vi "test Subset Pointer.vi"(8 "error in (no error)":errorcluster, 11 "TestCase in":refnum<class "Lifecycle Tests.lvclass">) -> (0 "error out":errorcluster, 3 "TestCase out":refnum<class "Lifecycle Tests.lvclass">)   [LabVIEW 2017, in "Pointer Tests.lvlib" / "Lifecycle Tests.lvclass"]
uses:
  Lifecycle Tests.lvclass
  Source/Classes/Pointer/Public/New/New (4B).vi
  Source/Classes/Pointer/Public/Write/Write (1D I32).vi
  Source/Classes/Pointer/Public/Read/Read (0D I32).vi
  Source/Classes/Pointer/Public/Write/Write (0D I32).vi
  <vilib>/addons/_JKI Toolkits/VI Tester/TestCase.llb/TestCase.lvclass
  Source/Classes/Pointer/Pointer.lvclass
  C:/Program Files (x86)/National Instruments/LabVIEW 2017/vi.lib/addons/_JKI Toolkits/VI Tester/TestCase.llb/TestCase.lvclass
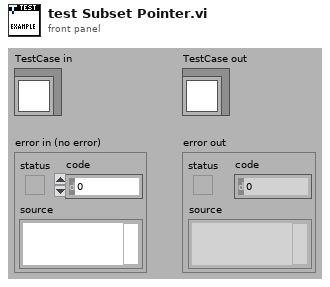
[diagram p1: front panel]
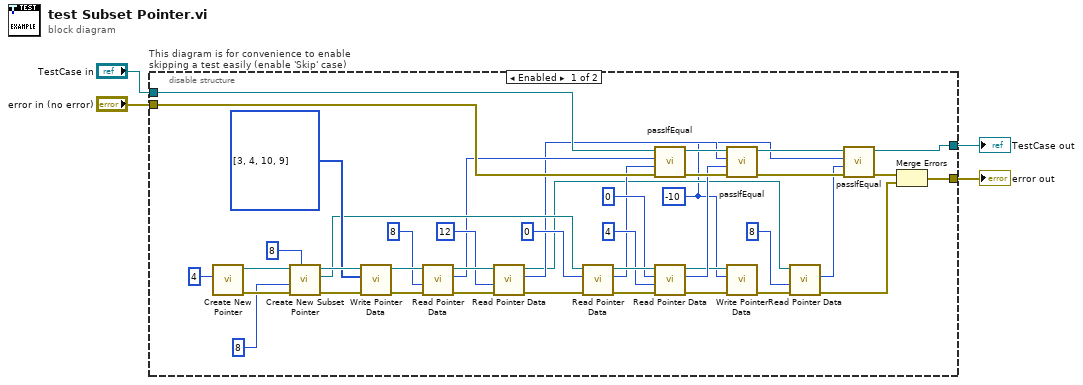
[diagram p0: block diagram]
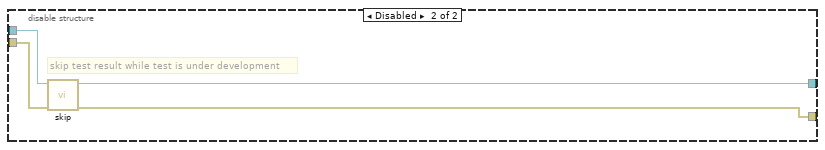
[diagram p2: hidden frame]
diagram:
  n1 = disable-structure "This diagram is for convenience to enable skipping a test easily (enable 'Skip' case)" shown="Enabled" {
    disable-tunnel: "TestCase in" -> [w23 w50]
    disable-tunnel: [w8 w48] -> w1
    disable-tunnel: [w16 w49] -> w3
    disable-tunnel: "error in (no error)" -> [w46 w47]
    frame Enabled {
      w7 = -10 ("length (-1: rest)")
      n2 = call-poly "Create New Pointer.vi"("count (1)"=u64 4) -> ("error out"=w40:errorcluster, "Pointer"=w45:refnum<class "Pointer.lvclass">)  [unwired: 9 in]
      n3 = call "Create New Subset Pointer.vi"("length (-1: rest)"=i64 8, "error in (no error)"=w40, "offset (0)"=u64 8, "base Pointer in"=w45) -> ("error out"=w33:errorcluster, "subset Pointer"=w38:refnum<class "Pointer.lvclass">, "base Pointer out"=w43:refnum<class "Pointer.lvclass">)  [unwired: 4 in, 1 out]
      n4 = call-poly "Write Pointer Data.vi"("error in (no error)"=w33, "buffer in"=i32[] [3, 4, 10, 9] ("length (-1: rest)"), "Pointer in"=w43) -> ("error out"=w39:errorcluster, "Pointer out"=w41:refnum<class "Pointer.lvclass">)  [unwired: 5 in, 2 out]
      n5 = call-poly "Read Pointer Data.vi"("error in (no error)"=w39, "offset (0)"=u64 8, "Pointer in"=w41) -> ("error out"=w32:errorcluster, "value out"=w20:i32, "Pointer out"=w26:refnum<class "Pointer.lvclass">)  [unwired: 5 in, 1 out]
      n6 = call-poly "Read Pointer Data.vi"("error in (no error)"=w32, "offset (0)"=u64 12, "Pointer in"=w26) -> ("error out"=w27:errorcluster, "value out"=w18:i32, "Pointer out"=w11:refnum<class "Pointer.lvclass">)  [unwired: 5 in, 1 out]
      n7 = call-poly "Read Pointer Data.vi"("error in (no error)"=w27, "value in"=0 ("length (-1: rest)"), "Pointer in"=w38) -> ("error out"=w30:errorcluster, "value out"=w19:i32, "Pointer out"=w31:refnum<class "Pointer.lvclass">)  [unwired: 5 in, 1 out]
      n8 = call-dynamic "passIfEqual.vi"("error in (no error)"=w46, "y"=w19, "x"=w20, "TestCase in"=w23) -> ("error out"=w24:errorcluster, "TestCase out"=w21:refnum<class "Lifecycle Tests.lvclass">)  [unwired: 6 in]
      n9 = call-poly "Read Pointer Data.vi"("error in (no error)"=w30, "offset (0)"=u64 4, "value in"=0 ("length (-1: rest)"), "Pointer in"=w31) -> ("error out"=w15:errorcluster, "value out"=w17:i32, "Pointer out"=w13:refnum<class "Pointer.lvclass">)  [unwired: 4 in, 1 out]
      n10 = call-dynamic "passIfEqual.vi"("error in (no error)"=w24, "y"=w17, "x"=w18, "TestCase in"=w21) -> ("error out"=w22:errorcluster, "TestCase out"=w9:refnum<class "Lifecycle Tests.lvclass">)  [unwired: 6 in]
      n11 = call-poly "Write Pointer Data.vi"("error in (no error)"=w15, "value"=w7, "Pointer in"=w13) -> ("error out"=w14:errorcluster)  [unwired: 5 in, 3 out]
      n12 = call-poly "Read Pointer Data.vi"("error in (no error)"=w14, "offset (0)"=u64 8, "Pointer in"=w11) -> ("error out"=w12:errorcluster, "value out"=w5:i32)  [unwired: 5 in, 2 out]
      n13 = call-dynamic "passIfEqual.vi"("error in (no error)"=w22, "y"=w5, "x"=w7, "TestCase in"=w9) -> ("error out"=w10:errorcluster, "TestCase out"=w8:refnum<class "Lifecycle Tests.lvclass">)  [unwired: 6 in]
      n14 = Merge Errors(w10, w12) -> (w16:errorcluster)
    }
    frame Disabled {
      # "skip test result while test is under development"
      n15 = call <vilib>:"skip.vi"("error in (no error)"=w47, "TestCase in"=w50) -> ("error out"=w49:errorcluster, "TestCase out"=w48:refnum<class "Lifecycle Tests.lvclass">)  [unwired: 8 in]
    }
  }
  "error out" <- w3
  "TestCase out" <- w1
